vi "Uint8Array Deserialize.vi"(8 "error in (no error)":errorcluster, 11 "Uint8Array DVR in":refnum<data-value>) -> (0 "error out":errorcluster, 2 "Data out":refnum<data-value>, 3 "Uint8Array DVR out":refnum<data-value>)   [LabVIEW 2010, in "MDSplus.lvlib"]
doc: "Returns the data as the result of a MDS deserialization of this byte array."
uses:
  <vilib>/MDSplus/Library/MDSplus.lvlib
  <vilib>/MDSplus/Classes/Data_Class/Array_Class/Uint8Array_Class/Uint8Array.lvclass
  <vilib>/MDSplus/Classes/Data_Class/Data.lvclass
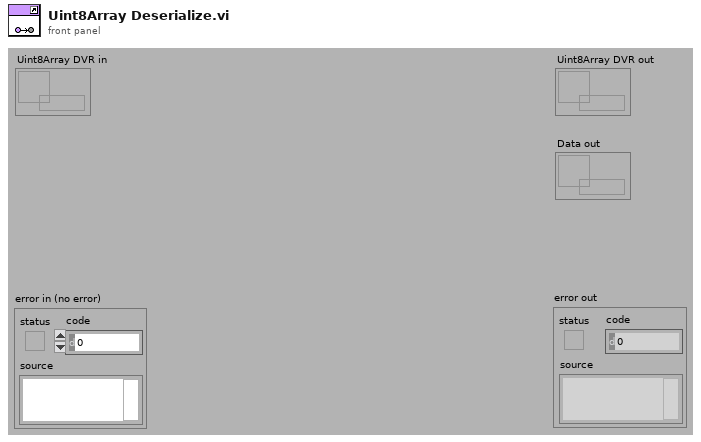
[diagram p1: front panel]
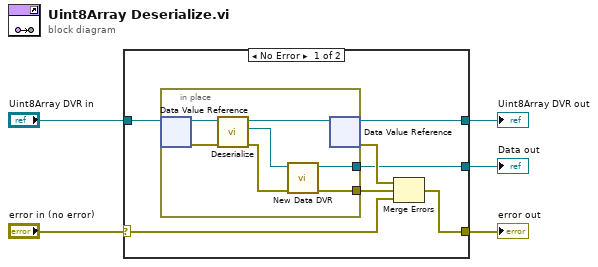
[diagram p0: block diagram]
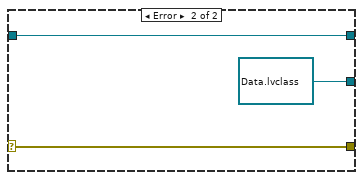
[diagram p2: hidden frame]
diagram:
  n1 = case shown="No Error" "error in (no error)" {
    selector: "error in (no error)" -> [w11 w22]
    tunnel: "Uint8Array DVR in" -> [w12 w21]
    tunnel: [w8 w22] -> w5
    tunnel: [w9 w21] -> w2
    tunnel: [w6 refnum<data-value> refnum ("Data DVR")] -> w1
    frame No Error {
      n2 = in-place {
        in-place-border: [w15] -> w6
        in-place-border: [w14] -> w7
        n3 = in-place-dvr #1(w12) -> (w19:refnum<class "Uint8Array.lvclass">, w18:errorcluster)
        n4 = call-dynamic "Deserialize.vi"("error in (no error)"=w18, "Uint8Array in"=w19) -> ("error out"=w13:errorcluster, "Data out"=w16:refnum<class "Data.lvclass">, "Uint8Array out"=w17:refnum<class "Uint8Array.lvclass">)  [unwired: 7 in]
        n5 = call <vilib>:"New Data DVR.vi"("error in (no error)"=w13, "Data in"=w16) -> ("error out"=w14:errorcluster, "Data DVR out"=w15:refnum<data-value>)  [unwired: 8 in]
        n6 = in-place-dvr #1(w17) -> (w9:refnum<data-value>, w10:errorcluster)
      }
      n7 = Merge Errors(w10, w7, w11) -> (w8:errorcluster)
    }
    frame Error {
    }
  }
  "error out" <- w5
  "Uint8Array DVR out" <- w2
  "Data out" <- w1
